vi "ParseSwerveModuleCancoder.vi"(8 "moduleName":string, 9 "configRef":T6) -> (2 "outputCluster":T1={"Sensor Initialization Strategy"=enum."Boot To Zero", "Absolute Sensor Range"=enum."Unsigned [0 to 360)", "Velocity Measurement Period"=100, "Velocity Measurement Window"=64, "Magnet Offset (Degrees)"=0.0, "Sensor Direction"=FALSE, "Sensor Coefficient"=0.087890625, "Unit String"="deg", "Sensor Time Base"=enum."PerMinute"} {"Velocity Measurement Period" items=["Period_1ms"=1, "Period_2ms"=2, "Period_5ms"=5, "Period_10ms"=10, "Period_20ms"=20, "Period_25ms"=25, "Period_50ms"=50, "Period_100ms"=100]; "Sensor Coefficient" format="%#_9g"}, 3 "configRefOut":T6)   [LabVIEW 2020]
uses:
  <vilib>/Utility/config.llb/Config Data RefNum.ctl
  <vilib>/Rock Robotics/WPI/ThirdParty/Phoenix-LabVIEW/CANCoder/Controls/CTRE_Phoenix_CANcoder_Configurables.ctl
  <vilib>/Rock Robotics/WPI/ThirdParty/Phoenix-LabVIEW/CANCoder/Controls/CTRE_Phoenix_CANcoder_SensorInitializationStrategy.ctl
  <vilib>/Rock Robotics/WPI/ThirdParty/Phoenix-LabVIEW/CANCoder/Controls/CTRE_Phoenix_CANcoder_AbsoluteSensorRange.ctl
  <vilib>/Rock Robotics/WPI/ThirdParty/Phoenix-LabVIEW/Motor Controller/Controls/CTRE_Phoenix_MotorControl_VelocityMeasurementPeriod.ctl
  <vilib>/Rock Robotics/WPI/ThirdParty/Phoenix-LabVIEW/CANCoder/Controls/CTRE_Phoenix_CANcoder_SensorTimeBase.ctl
  <vilib>/Utility/config.llb/Read Key (I32).vi
  <vilib>/Utility/config.llb/Read Key (Boolean).vi
  <vilib>/Utility/config.llb/Read Key (Double).vi
  <vilib>/Utility/config.llb/NI_LVConfig.lvlib
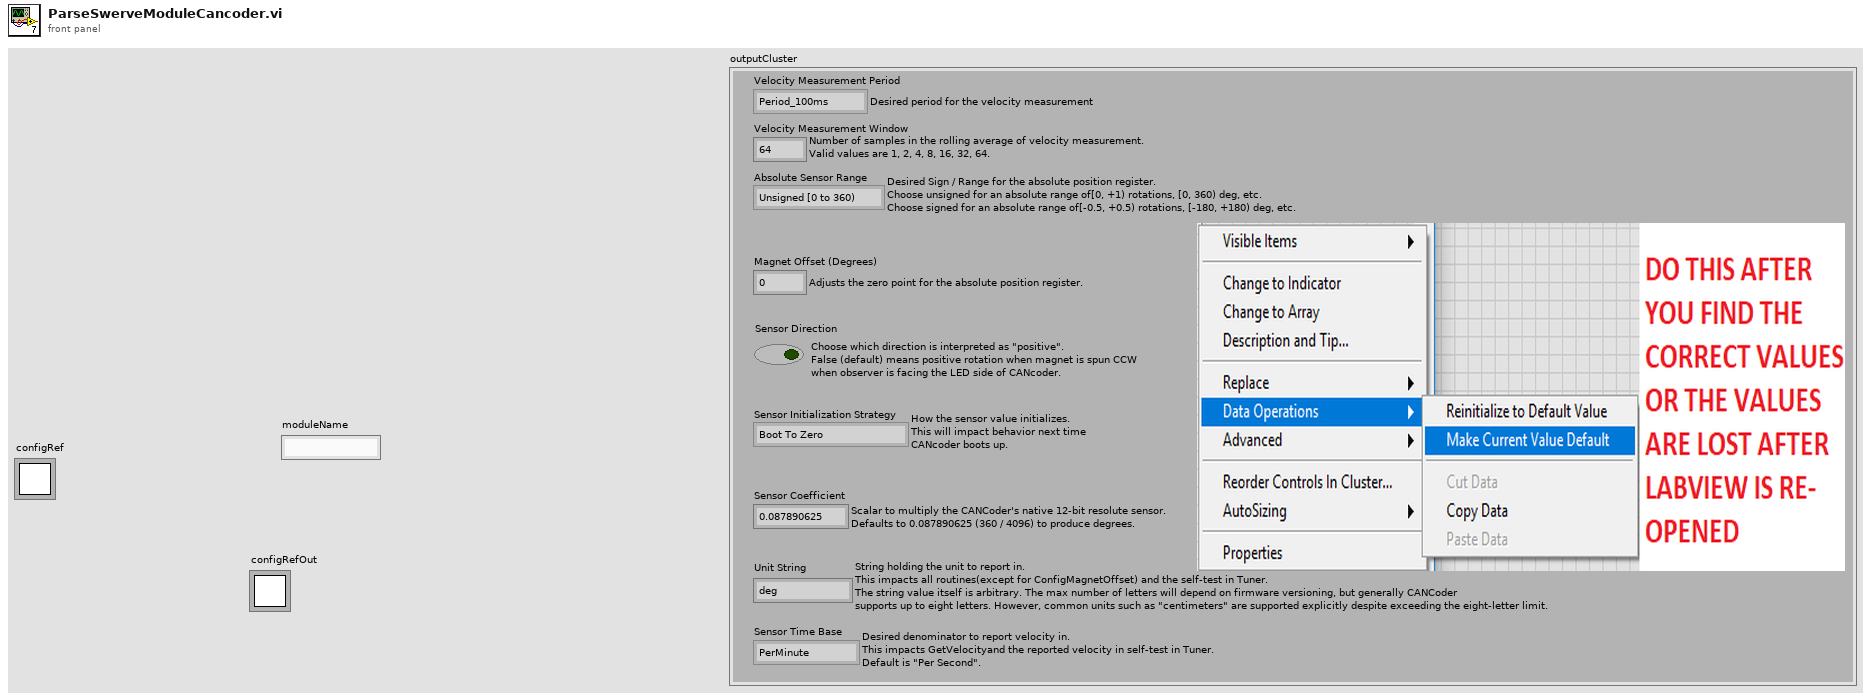
[diagram p1: front panel]
types:
  T1 = typedef "CTRE_Phoenix_CANcoder_Configurables.ctl" = cluster{"Sensor Initialization Strategy":T2, "Absolute Sensor Range":T3, "Velocity Measurement Period":T4, "Velocity Measurement Window":i32, "Magnet Offset (Degrees)":dbl, "Sensor Direction":bool, "Sensor Coefficient":dbl, "Unit String":string, "Sensor Time Base":T5}
  T2 = typedef "CTRE_Phoenix_CANcoder_SensorInitializationStrategy.ctl" = enum16{"Boot To Zero", "Boot To Absolute Position"}
  T3 = typedef "CTRE_Phoenix_CANcoder_AbsoluteSensorRange.ctl" = enum16{"Unsigned [0 to 360)", "Signed [-180 to +180)"}
  T4 = typedef "CTRE_Phoenix_MotorControl_VelocityMeasurementPeriod.ctl" = u16
  T5 = typedef "CTRE_Phoenix_CANcoder_SensorTimeBase.ctl" = enum16{"Per100Ms_Legacy", "PerSecond", "PerMinute"}
  T6 = typedef "NI_LVConfig.lvlib/Config Data RefNum.ctl" = refnum<k1>
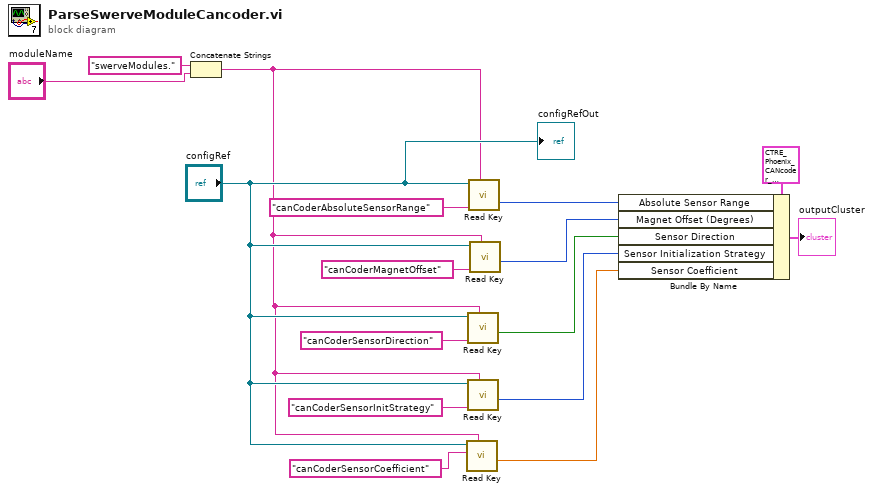
[diagram p0: block diagram]
diagram:
  n1 = Concatenate Strings("swerveModules." ("string"), "moduleName") -> (w2:string)
  n2 = call-poly <vilib>:"Read Key.vi"("section"=w2, "key"="canCoderSensorCoefficient", "refnum"="configRef") -> ("value"=w4:dbl)  [unwired: 5 in, 3 out]
  n3 = call-poly <vilib>:"Read Key.vi"("section"=w2, "key"="canCoderSensorDirection", "refnum"="configRef") -> ("value"=w10:bool)  [unwired: 5 in, 3 out]
  n4 = call-poly <vilib>:"Read Key.vi"("section"=w2, "key"="canCoderSensorInitStrategy", "refnum"="configRef") -> ("value"=w8:i32)  [unwired: 5 in, 3 out]
  n5 = call-poly <vilib>:"Read Key.vi"("section"=w2, "key"="canCoderAbsoluteSensorRange", "refnum"="configRef") -> ("value"=w6:i32)  [unwired: 5 in, 3 out]
  n6 = call-poly <vilib>:"Read Key.vi"("section"=w2, "key"="canCoderMagnetOffset", "refnum"="configRef") -> ("value"=w12:i32)  [unwired: 5 in, 3 out]
  n7 = Bundle By Name(cluster=T1 {"Sensor Initialization Strategy"=enum."Boot To Zero", "Absolute Sensor Range"=enum."Unsigned [0 to 360)", "Velocity Measurement Period"=100, "Velocity Measurement Window"=64, "Magnet Offset (Degrees)"=0.0, "Sensor Direction"=FALSE, "Sensor Coefficient"=0.087890625, "Unit String"="deg", "Sensor Time Base"=enum."PerMinute"} ("cancoderConfig"), "Absolute Sensor Range"=w6, "Magnet Offset (Degrees)"=w12, "Sensor Direction"=w10, "Sensor Initialization Strategy"=w8, "Sensor Coefficient"=w4) -> (→"outputCluster":T1)
  "configRefOut" <- "configRef"
